vi "read_log.vi"() -> ()   [LabVIEW 2013]
uses:
  Data/TypeDefs/Log_Data.ctl
  Data/TypeDefs/Notifiers.ctl
  Data/TypeDefs/UTM Location.ctl
  Data/TypeDefs/Sail Set Suggestions.ctl
  Data/TypeDefs/Rudder Set Suggestions.ctl
  Data/TypeDefs/OverrideInformation.ctl
  Data/TypeDefs/OverrideMode.ctl
  Data/TypeDefs/MotorSetup.ctl
  Data/TypeDefs/DynamixelSetupInfo.ctl
  Data/TypeDefs/AirmarStatus.ctl
  Data/TypeDefs/HardwareOnline.ctl
  Data/TypeDefs/DynamixelCycleTracker.ctl
  Data/TypeDefs/RC Input Values.ctl
  Logic/Classes/Waypoint/Waypoint.lvclass
panel:
  out "Array 2":string[](array[string])
  out "Array":string[](array[string])
  out "size(s)":i32
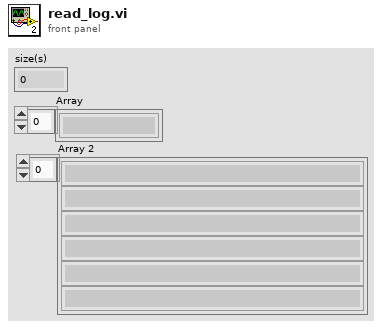
[diagram p1: front panel]
types:
  T1 = typedef "Log_Data.ctl" = cluster{"names":string, "value":variant}
  T2 = typedef "Notifiers.ctl" = cluster{"BoatSpeed":refnum<notifier>, "WindSpeed":refnum<notifier>, "EStop":refnum<notifier>, "BoatDirection":refnum<notifier>, "Luffing":refnum<notifier>, "RudderForce":refnum<notifier>, "BatteryVoltage":refnum<notifier>, "StayForces":refnum<notifier>, "BoatLocation":refnum<notifier>, "Pitch":refnum<notifier>, "Roll":refnum<notifier>, "RateOfTurn":refnum<notifier>, "RelWindDirection":refnum<notifier>, "SailPositions":refnum<notifier>, "RudderPosition":refnum<notifier>, "IronsRange":refnum<notifier>, "AbsWindDirection":refnum<notifier>, "OverrideInformation":refnum<notifier>, "DynamixelTorques":refnum<notifier>, "MotorSetup":refnum<notifier>, "AirmarStatus":refnum<notifier>, "HardwareOnline?":refnum<notifier>, "Sim_ActualSailPositions [0,1]":refnum<notifier>, "DynamixelCycleTracker":refnum<notifier>, "BoatVelocityDirection":refnum<notifier>, "SimWindHeading(rad)":refnum<notifier>, "SimWindSpeed(m/s)":refnum<notifier>, "RCInputValues":refnum<notifier>, "Finished Waypoints":refnum<notifier>, "DesiredHeading":refnum<notifier>, "Latest Mission ID":refnum<notifier>, "Latest Obstacle ID":refnum<notifier>, "DownwindDiscouragedRange":refnum<notifier>, "Tack Range":refnum<notifier>}
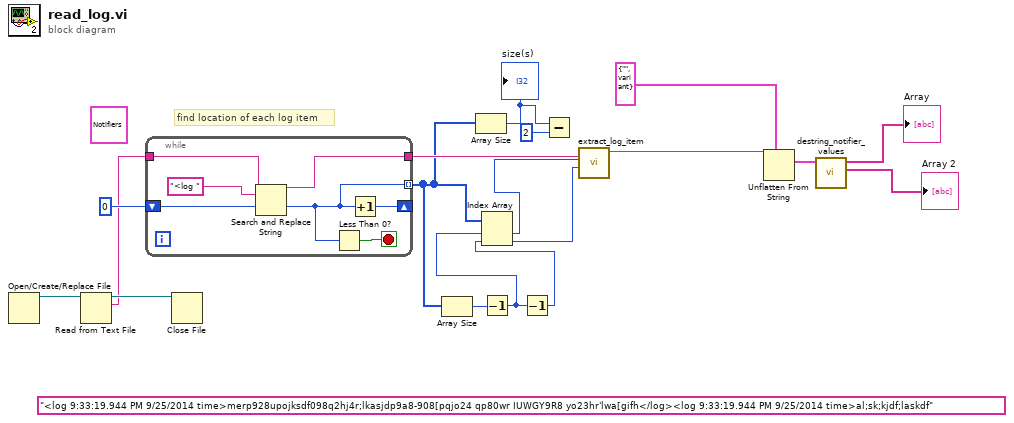
[diagram p0: block diagram]
diagram:
  (unwired) "<log 9:33:19.944 PM 9/25/2014 time>merp928upojksdf098q2hj4r;lkasjdp9a8-908[pqjo24 qp80wr IUWGY9R8 yo23hr'lwa[gifh</log><log 9:33:19.944 PM 9/25/2014 time>al;sk;kjdf;laskdf"
  (unwired) T2 {"BoatSpeed"=refnum, "WindSpeed"=refnum, "EStop"=refnum, "BoatDirection"=refnum, "Luffing"=refnum, "RudderForce"=refnum, "BatteryVoltage"=refnum, "StayForces"=refnum, "BoatLocation"=refnum, "Pitch"=refnum, "Roll"=refnum, "RateOfTurn"=refnum, "RelWindDirection"=refnum, "SailPositions"=refnum, "RudderPosition"=refnum, "IronsRange"=refnum, "AbsWindDirection"=refnum, "OverrideInformation"=refnum, "DynamixelTorques"=refnum, "MotorSetup"=refnum, "AirmarStatus"=refnum, "HardwareOnline?"=refnum, "Sim_ActualSailPositions [0,1]"=refnum, "DynamixelCycleTracker"=refnum, "BoatVelocityDirection"=refnum, "SimWindHeading(rad)"=refnum, "SimWindSpeed(m/s)"=refnum, "RCInputValues"=refnum, "Finished Waypoints"=refnum, "DesiredHeading"=refnum, "Latest Mission ID"=refnum, "Latest Obstacle ID"=refnum, "DownwindDiscouragedRange"=refnum, "Tack Range"=refnum} ("NotifierReferences")
  # "find location of each log item"
  n1 = Open/Create/Replace File() -> (refnum out=w12:refnum<file>)  [unwired: 6 in, 2 out]
  n2 = Read from Text File(file (use dialog)=w12) -> (refnum out=w13:refnum<file>, text=w11:string)  [unwired: 3 in, 2 out]
  n3 = while {
    tunnel: w11 -> [w25]
    shift-right: [w19] -> _
    shift-left: 0 ("offset past replacement") -> [w21]
    tunnel: [w22] -> w16
    tunnel: [w20] -> w4 mode=indexing
    stop <- w23 stop-if-true
    n4 = Search and Replace String(input string=w25, search string="<log ", offset=w21) -> (result string=w22:string, offset past replacement=w20:i32)  [unwired: 5 in, 2 out]
    n5 = Less Than 0?(x=w20) -> (x < 0?=w23:bool)
    n6 = Increment(x=w20) -> (x+1=w19:i32)
  }
  n7 = Close File(refnum=w13) -> ()  [unwired: 1 in, 2 out]
  n8 = Array Size(array=w4) -> (size(s)=w3:i32)
  n9 = Array Size(array=w4) -> (size(s)=w5:i32)
  "size(s)" <- w5
  n10 = Decrement(x=w3) -> (x-1=w2:i32)
  n11 = Decrement(x=w2) -> (x-1=w1:i32)
  n12 = Index Array(array=w4, index #1=w2, index #2=w1) -> (element #1=w15:i32, element #2=w14:i32)
  n13 = Subtract(x=w5, y=2) -> ()  [unwired: 1 out]
  n14 = call "extract_log_item.vi"("next location"=w14, "location"=w15, "full string"=w16) -> ("message"=w7:string)  [unwired: 7 in, 1 out]
  n15 = Unflatten From String(type=T1 {"names"="", "value"=variant} ("input cluster"), binary string=w7) -> (value=w6:T1)  [unwired: 3 in, 2 out]
  n16 = call "destring_notifier_values.vi"("input cluster 2"=w6) -> ("Array 2"=→"Array 2":string[], "Array"=→"Array":string[])  [unwired: 9 in]
